vi "ParseSysexAnalogMapping.vi"(8 "error in":errorcluster, 11 "Sysex Message":u8[](array[numeric]) format="%x") -> (0 "error out":errorcluster, 1 "IsValidSysex":bool, 3 "AnalogChannels":dbl[](array[numeric]))   [LabVIEW 2020, in "FirmataClient.lvlib"]
doc: "Parse a message according to the Firmata Protocol Requirements. \n- https://github.com/firmata/protocol\n- https://github.com/firmata/protocol/blob/master/protocol.md"
uses:
  FirmataClient.lvlib
  controls/FGV-Mode.ctl
  controls/FirmataProtocolConstants.ctl
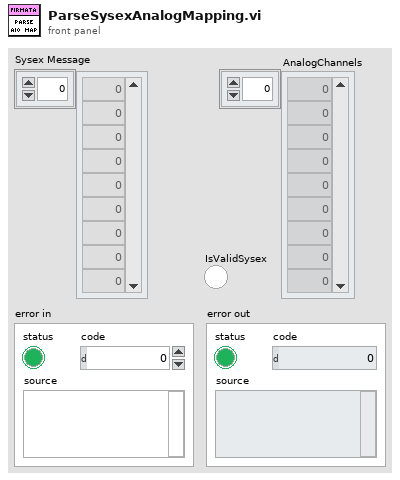
[diagram p1: front panel]
types:
  T1 = typedef "FirmataClient.lvlib/FirmataProtocolConstants.ctl" = u16
  T2 = typedef "FirmataClient.lvlib/FGV-Mode.ctl" = enum16{"Load Comport", "Load Board Capabilities", "Read"}
  T3 = typedef "FirmataClient.lvlib/PinModesListData.ctl" = cluster{"DigitalInputMode":T4, "DigitalOutputMode":T4, "AnalogInputMode":T4, "PWMMode":T4, "ServoMode":T4, "ShiftMode":T4, "I2CMode":T4, "OneWireMode":T4, "StepperMode":T4, "EncoderMode":T4, "SerialMode":T4, "InputPullupMode":T4, "Ext.SPIMode":T4, "Ext.SonarMode":T4, "Ext.ToneMode":T4, "Ext.DHTMode":T4, "Index":cluster{"DigitalIndex":u16, "AnalogIndex":dbl}}
  T4 = typedef "FirmataClient.lvlib/PinModeData.ctl" = cluster{"Resolution":u8, "btn":bool, "PinMode":T5}
  T5 = typedef "FirmataClient.lvlib/FirmataPinModes.ctl" = enum16{"DigitalInput", "DigitalOutput", "AnalogInput", "PWM", "Servo", "Shift", "I2C", "OneWire", "Stepper", "Encoder", "Serial", "InputPullup", "Extended.SPI", "Extended.Sonar", "Extended.Tone", "Extended.DHT"}
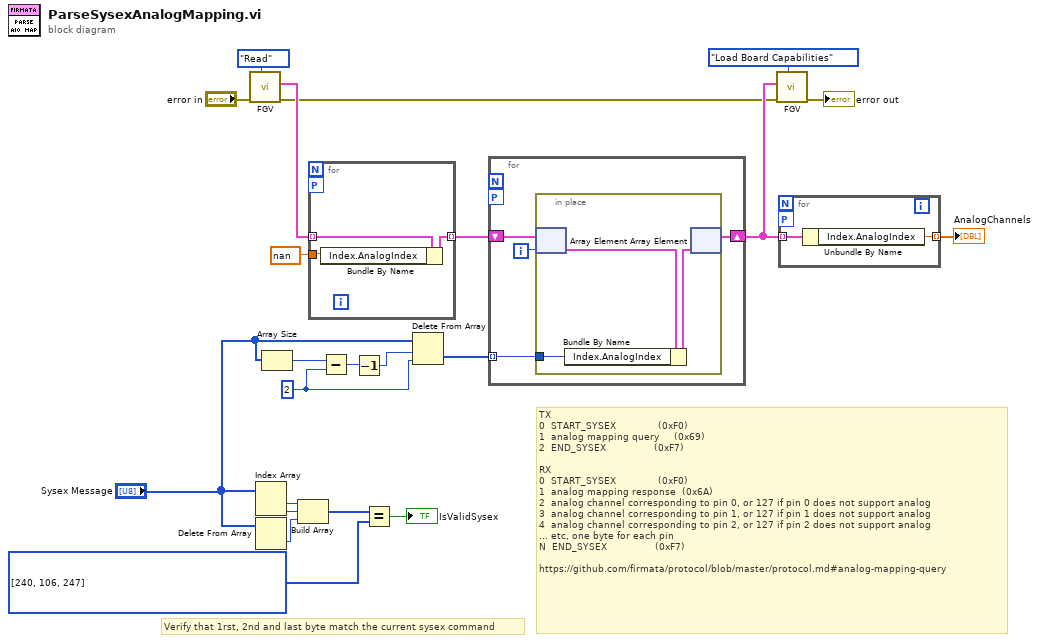
[diagram p0: block diagram]
diagram:
  w4 = T1[] [240, 106, 247] items=["ANALOG_IO_MESSAGE"=224, "DIGITAL_IO_MESSAGE"=144, "REPORT_ANALOG_PIN"=192, "REPORT_DIGITAL_PORT"=208, "START_SYSEX"=240, "END_SYSEX"=247, "SET_PIN_MODE"=244, "SET_DIGITAL_PIN_VALUE"=245, "PROTOCOL_VERSION"=249, "SYSTEM_RESET"=255, "SYSEX.EXTENDED_ID"=0, "SYSEX.RESERVED_USER_COMMANDs"=1, "SYSEX.ANALOG_MAPPING_QUERY"=105, "SYSEX.ANALOG_MAPPING_RESPONSE"=106, "SYSEX.CAPABILITY_QUERY"=107, "SYSEX.CAPABILITY_RESPONSE"=108, "SYSEX.PIN_STATE_QUERY"=109, "SYSEX.PIN_STATE_RESPONSE"=110, "SYSEX.REPORT_FIRMWARE"=121, "SYSEX.EXTENDED_ANALOG"=111, "SYSEX.STRING_DATA"=113, "SYSEX.REALTIME"=127, "SYSEX.NON_REALTIME"=126, "SYSEX.SAMPLING_INTERVAL"=122]
  w13 = 2 ("index")
  # "Verify that 1rst, 2nd and last byte match the current sysex command"
  # "TX\n0  START_SYSEX              (0xF0)\n1  analog mapping query     (0x69)\n2  END_SYSEX                (0xF7)\n\nRX\n0  START_SYSEX              (0xF0)\n1  analog mapping response  (0x6A)\n2  analog channel corresponding to pin 0, or 127 if pin 0 does not support analog\n3  analog channel corresponding to pin 1, or 127 if pin 1 does not support analog\n4  analog channel corresponding to pin 2, or 127 if pin 2 does not support analog\n... etc, one byte for each pin\nN  END_SYSEX                (0xF7)\n\nhttps://github.com/firmata/protocol/blob/master/protocol.md#analog-mapping-query"
  n1 = call "FGV.vi"("Mode"=FGV-Mode."Read", "error in"="error in") -> ("error out"=w2:errorcluster, "Board Pins Out"=w8:T3[])  [unwired: 7 in, 1 out]
  n2 = Index Array(array="Sysex Message") -> (element #1=w22:u8, element #2=w20:u8)  [unwired: 2 in]
  n3 = Delete From Array(array="Sysex Message") -> (deleted portion=w21:u8)  [unwired: 2 in, 1 out]
  n4 = Array Size(array="Sysex Message") -> (size(s)=w14:i32)
  n5 = Build Array(w22, w20, w21) -> (w19:u8[])
  n6 = for {
    tunnel: [w24] -> w9 mode=indexing
    tunnel: w8 -> [w25] mode=indexing
    tunnel: nan ("AnalogChannel") -> [w23]
    workers-P: _ -> [_]
    n7 = Bundle By Name(cluster=w25, "Index.AnalogIndex"=w23) -> (w24:T3)
  }
  n8 = Subtract(x=w14, y=w13) -> (x-y=w12:i32)
  n9 = Decrement(x=w12) -> (x-1=w11:i32)
  n10 = Equal?(x=w19, y=w4) -> (x = y?=→"IsValidSysex":bool)
  n11 = Delete From Array(array="Sysex Message", length=w11, index=w13) -> (deleted portion=w10:u8[])  [unwired: 1 out]
  n12 = for {
    shift-right: [w29] -> w6
    shift-left: w9 -> [w26]
    tunnel: w10 -> [w27] mode=indexing
    workers-P: _ -> [_]
    i -> [w28]
    n13 = in-place {
      in-place-border: w27 -> [w31]
      n14 = in-place-array #1(w26, w28) -> (w32:T3)
      n15 = Bundle By Name(cluster=w32, "Index.AnalogIndex"=w31) -> (w30:T3)
      n16 = in-place-array #1(w30) -> (w29:T3[])  [unwired: 1 out]
    }
  }
  n17 = call "FGV.vi"("Mode"=FGV-Mode."Load Board Capabilities", "error in"=w2, "Board Pins In"=w6) -> ("error out"=→"error out":errorcluster)  [unwired: 6 in, 2 out]
  n18 = for {
    tunnel: w6 -> [w34] mode=indexing
    tunnel: [w33] -> w5 mode=indexing
    workers-P: _ -> [_]
    n19 = Unbundle By Name(w34) -> ("Index.AnalogIndex"=w33:dbl)
  }
  "AnalogChannels" <- w5
